vi "PWM_Motor_Überholen.vi"(1 "Abstand Bande erreicht":bool, 7 "Sensor geradeaus rechts":dbl, 9 "Sensor geradeaus links":dbl, 11 "Motor folgen":dbl) -> (4 "PWM Motor":dbl=0.3)   [LabVIEW 2016]
doc: "Geschwindigkeitsregelung anhand IR Sensor vorne\n05.04.17_Tloe"
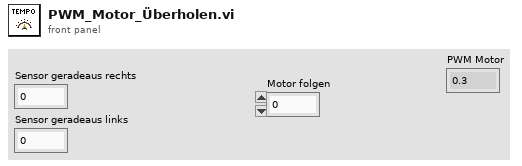
[diagram p1: front panel]
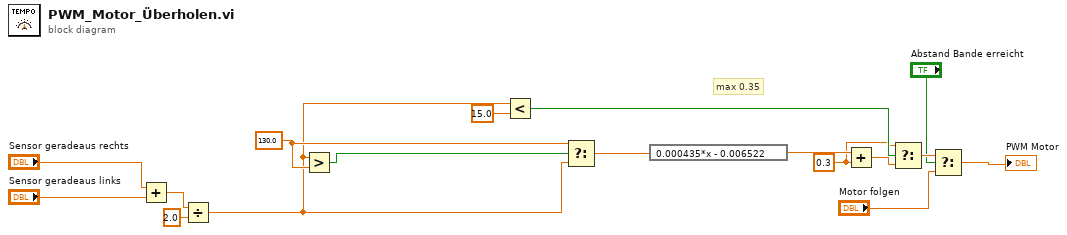
[diagram p0: block diagram]
diagram:
  w2 = 0.3 ("y")
  w8 = 130.0 ("y")
  # "max 0.35"
  n1 = Add(x="Sensor geradeaus rechts", y="Sensor geradeaus links") -> (x+y=w15:dbl)
  n2 = Divide(x=w15, y=2.0) -> (x/y=w7:dbl)
  n3 = Greater?(x=w7, y=w8) -> (0:w9:bool)
  n4 = Less?(x=w7, y=15.0) -> (x < y?=w3:bool)
  n5 = Select(t=w8, s=w9, f=w7) -> (s? t:f=w11:dbl)
  n6 = expression code="0.000435*x - 0.006522"(w11) -> (w10:dbl)
  n7 = Add(x=w10, y=w2) -> (x+y=w4:dbl)
  n8 = Select(t=w2, s=w3, f=w4) -> (s? t:f=w5:dbl)
  n9 = Select(t=w5, s="Abstand Bande erreicht", f="Motor folgen") -> (s? t:f=→"PWM Motor":dbl)
